vi "Module Init.vi"(8 "error in (no error)":errorcluster, 11 "Role Manager in":refnum<class "Role Manager.lvclass">) -> (0 "error out":errorcluster, 3 "Role Manager out":refnum<class "Role Manager.lvclass">)   [LabVIEW 2020, in "Volatus.lvlib" / "Role Manager.lvclass"]
uses:
  Role Manager.lvclass
  Role Manager.lvclass/Role Manager.ctl
  Module/Module.lvclass
  C:/dev/lv20CE/relink/lv-volatus/Volatus/Module/Module.lvclass
  C:/dev/lv20CE/relink/lv-volatus/Volatus/Role Manager/Role Manager.lvclass
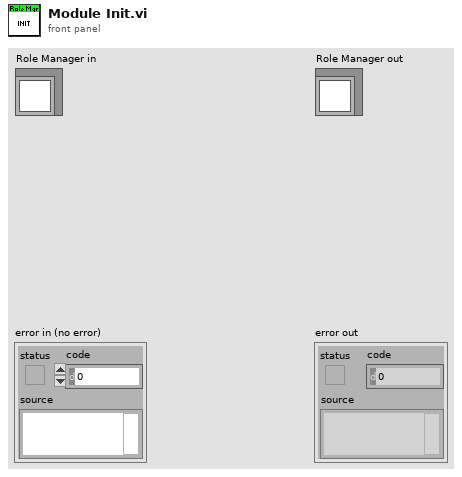
[diagram p1: front panel]
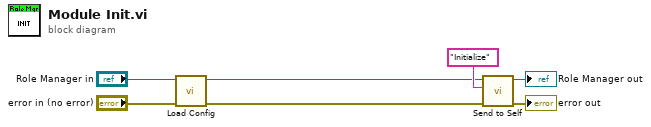
[diagram p0: block diagram]
diagram:
  n1 = call "Load Config.vi"("error in (no error)"="error in (no error)", "Role Manager in"="Role Manager in") -> ("error out"=w3:errorcluster, "Role Manager out"=w1:refnum<class "Role Manager.lvclass">)  [unwired: 8 in]
  n2 = call "Send to Self.vi"("error in (no error)"=w3, "Message ID"="Initialize", "Module in"=w1) -> ("error out"=→"error out":errorcluster, "Module in"=→"Role Manager out":refnum<class "Role Manager.lvclass">)  [unwired: 7 in]
